vi "To908.vi"(11 "In":string) -> (3 "Out":string)   [LabVIEW 2011]
panel:
  # "To908.vi\nPassword:Abcd1234*\n20221117:Start new version for build Short project name to project908"
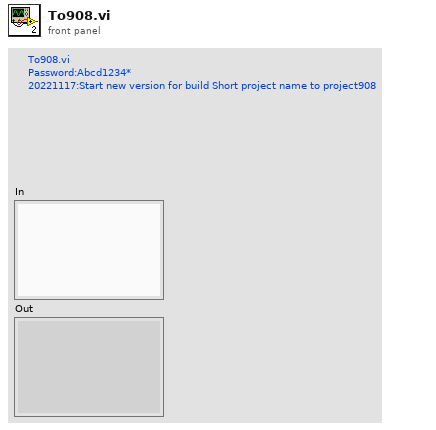
[diagram p1: front panel]
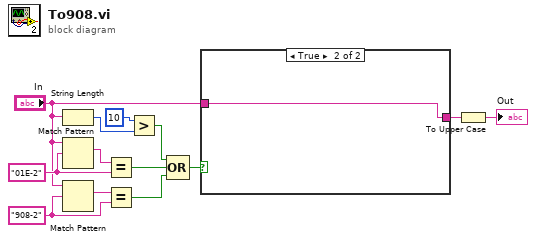
[diagram p0: block diagram]
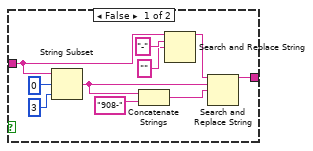
[diagram p2: hidden frame]
diagram:
  w9 = "01E-2" ("regular expression")
  w11 = "908-2" ("regular expression")
  n1 = String Length(string="In") -> (length=w2:i32)
  n2 = Match Pattern(string="In", regular expression=w9) -> (match substring=w10:string)  [unwired: 1 in, 3 out]
  n3 = Match Pattern(string="In", regular expression=w11) -> (match substring=w12:string)  [unwired: 1 in, 3 out]
  n4 = Equal?(x=w10, y=w9) -> (x = y?=w6:bool)
  n5 = Equal?(x=w12, y=w11) -> (x = y?=w7:bool)
  n6 = Greater?(x=10, y=w2) -> (0:w5:bool)
  n7 = Compound Arithmetic op=OR(w5, w6, w7) -> (w4:bool)
  n8 = case shown="True" w4 {
    tunnel: "In" -> [w20 w24]
    tunnel: [w14 w24] -> w13
    frame False {
      n9 = String Subset(string=w20, offset (0)=0, length (rest)=3 ("length (rest)")) -> (substring=w17:string)
      n10 = Concatenate Strings(w17, "908-" ("string")) -> (w15:string)
      n11 = Search and Replace String(input string=w20, search string="-", replace string="" ("replace string (\"\")")) -> (result string=w21:string)  [unwired: 5 in, 3 out]
      n12 = Search and Replace String(input string=w21, search string=w17, replace string=w15) -> (result string=w14:string)  [unwired: 5 in, 3 out]
    }
    frame True {
    }
  }
  n13 = To Upper Case(1:w13) -> (0:→"Out":string)
